vi "32xx_Config_RS232.vi"(4 "Serial_Settings.ctltermination char\n(0xA = '\\n' = LF)":u8=13 format="%x", 6 "Enable Termination\nChar (F)":bool, 7 "Taille buffers E/S":u32=64, 8 "entrée d'erreur":errorcluster caption="entrée d'erreur (pas d'erreur)", 9 "Paramètres série":T1={"Bauds"=9600, "bits"=8, "     Parité :"=enum."None", "bit(s) de stop"=10, "CTRL flux"=0} {"CTRL flux" items=["Aucun(e)"=0, "XON/XOFF"=1, "RTS/CTS"=2, "DTR/DSR"=4]; "bit(s) de stop" items=["1.0"=10, "2.0"=20]; "bits" min=5 max=8 step=1; "Bauds" items=["75"=75, "110"=110, "134"=134, "150"=150, "300"=300, "600"=600, "1200"=1200, "1800"=1800, "2400"=2400, "4800"=4800, "7200"=7200, "9600"=9600, "14400"=14400, "19200"=19200, "28800"=28800, "38400"=38400, "56000"=56000, "57600"=57600, "115200"=115200, "128000"=128000, "230400"=230400]}, 10 "TimeOut (ms)":u32=6500, 11 "Port Entrée":refnum<visa-resource-name>="COM1") -> (0 "sortie d'erreur":errorcluster, 3 "Port Sortie":refnum<visa-resource-name>="COM1")   [LabVIEW 2020]
doc: "Configuration du port COM en RS232 : Baud rate, data bits ; etc.."
panel:
  # "© 2008 2020 elc  ALL RIGHTS RESERVED."
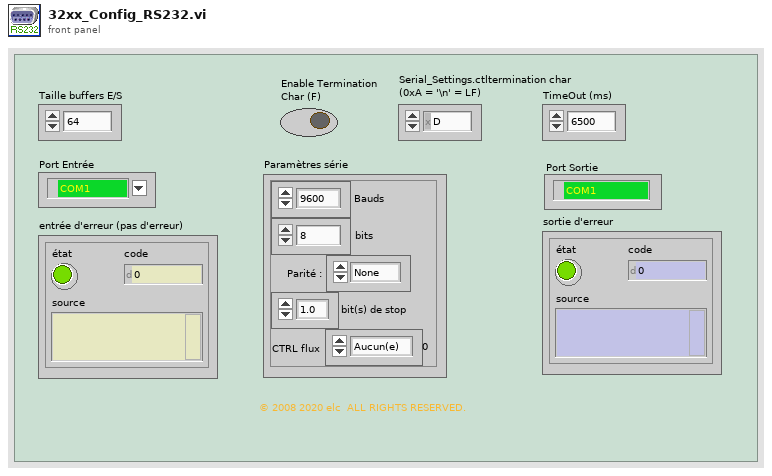
[diagram p1: front panel]
types:
  T1 = cluster{"Bauds":u32, "bits":u16, "     Parité :":enum16{"None", "Odd", "Even", "Mark", "Space"}, "bit(s) de stop":u16, "CTRL flux":u16}
  T2 = typedef "32xx_VISA_Flush_IO_BuffMask_Custom.ctl" = u16
  T3 = typedef "32xx_VISA_Set_IO_Buffer_Mask_Custom.ctl" = u16
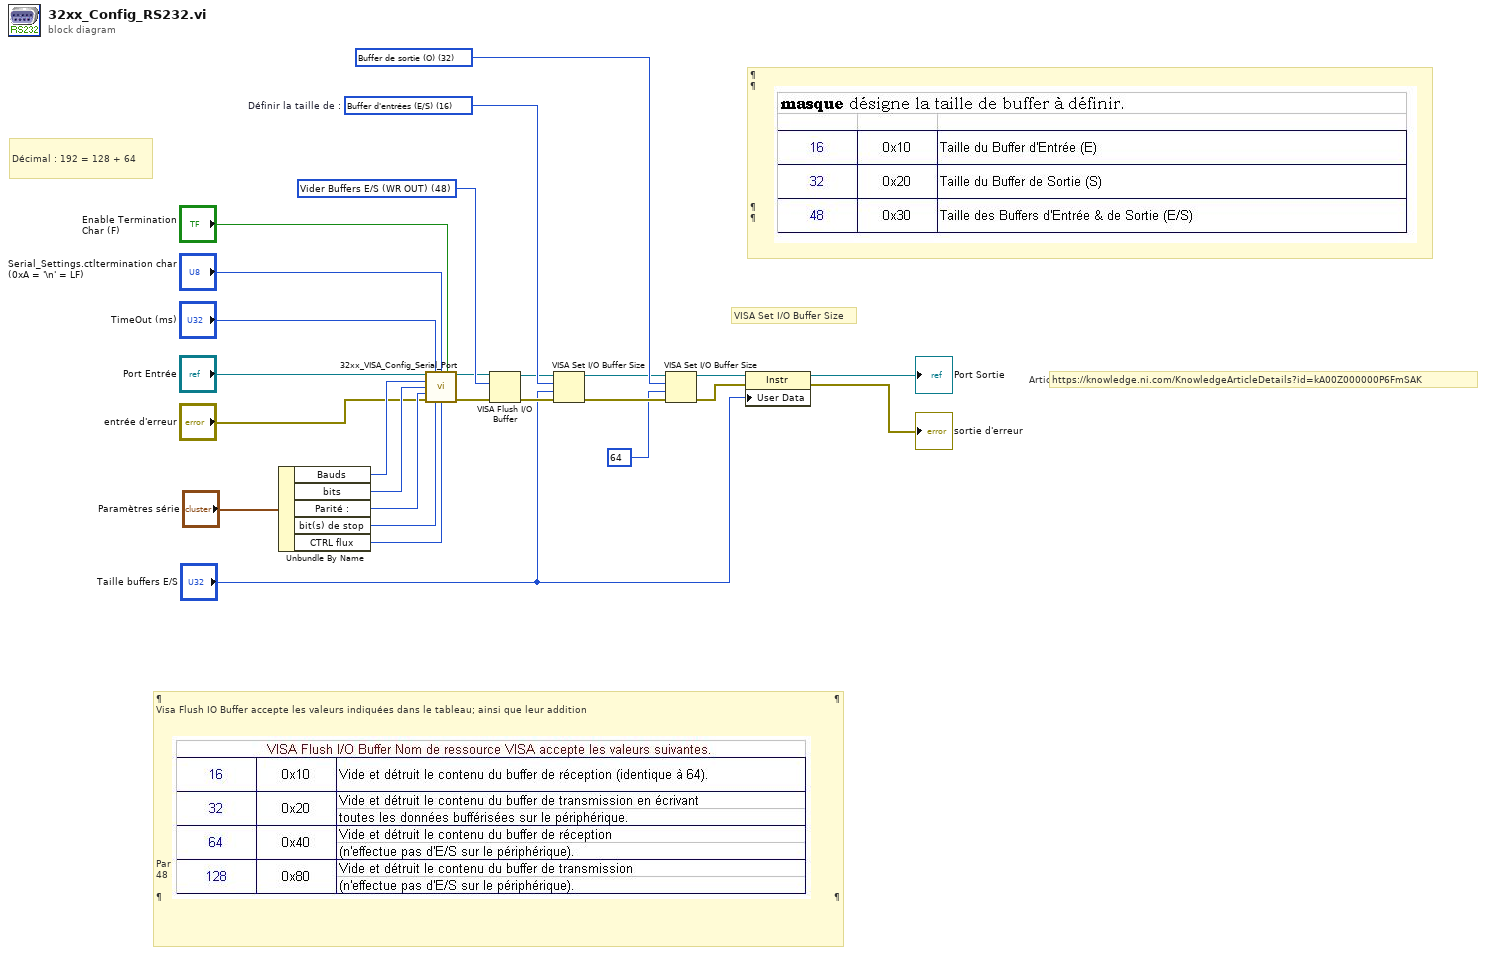
[diagram p0: block diagram]
diagram:
  w19 = T2 48 items=["Vider le buffer d'entrée"=16, "Écrire le buffer de sortie sur le périphérique"=32, "Vider Buffers E/S (WR OUT)"=48, "Vider le buffer d'entrée (Pas d'E/S)"=64, "Vider le buffer de sortie  (sans écrire)"=128, "Vider les buffers E/S  (Pas d'E/S)"=192] ("Mask")
  w22 = T3 32 items=["Buffer d'entrée (I)"=16, "Buffer de sortie (O)"=32, "Buffer d'entrée et de sorties (I/O)"=48] ("Mask")
  w26 = T3 16 items=["Buffer d'entrées (E/S)"=16, "Buffer de sorties (E/S)"=32, "Buffers d'entrées et de sorties (E/S)"=48]  # Définir la taille de :
  # "https://knowledge.ni.com/KnowledgeArticleDetails?id=kA00Z000000P6FmSAK"
  # "Article de labView au sujet  de l'erreur  -1073807298 & du Flush automatique :"
  # "VISA Set I/O Buffer Size"
  # "Décimal : 192 = 128 + 64"
  # "¶                                                                                                                                                                                                                               ¶\n\n\n\n\n\n\n\n\n\n\n¶                                                                                                                                                                                                                               ¶"
  # "¶                                                                                                                                                                                                                                ¶\nVisa Flush IO Buffer accepte les valeurs indiquées dans le tableau; ainsi que leur addition\n\n\n\n\n\n\n\n\n\n\n\n\n\nPar exemple, la valeur 192 (0xC0 = 0x40 + 0x80)  videra les buffers d'entrée & de sortie, sans écrire sur le périphérique.\n48 = 0x30 = 0x10 + 0x20\n\n¶                                                                                                                                                                                                                                ¶"
  n1 = Unbundle By Name("Paramètres série") -> ("Bauds"=w11:u32, "bits"=w10:u16, "Parité :"=w9:enum16{"None", "Odd", "Even", "Mark", "Space"}, "bit(s) de stop"=w4:u16, "CTRL flux"=w3:u16)
  n2 = call "32xx_VISA_Config_Serial_Port.vi"("VISA resource name"="Port Entrée", "timeout (10sec)"="TimeOut (ms)", "termination char\n(0xA = '\\n' = LF)"="Serial_Settings.ctltermination char\n(0xA = '\\n' = LF)", "Enable Termination\nChar (T)"="Enable Termination\nChar (F)", "baud rate (9600)"=w11, "data bits (8)"=w10, "parity (0:none)"=w9, "error in (no error)"="entrée d'erreur", "stop bits (10: 1 bit)"=w4, "flow control (0:none)"=w3) -> ("référence en sortie"=w1:refnum<visa-resource-name>, "error out"=w2:errorcluster)  [unwired: 4 in]
  n3 = VISA Flush I/O Buffer(VISA resource name=w1, mask (16)=w19, error in (no error)=w2) -> (VISA resource name out=w24:refnum<visa-resource-name>, error out=w23:errorcluster)
  n4 = VISA Set I/O Buffer Size(VISA resource name=w24, mask (16)=w26, size (4096)="Taille buffers E/S", error in (no error)=w23) -> (VISA resource name out=w21:refnum<visa-resource-name>, error out=w20:errorcluster)
  n5 = VISA Set I/O Buffer Size(VISA resource name=w21, mask (16)=w22, size (4096)=u32 64 ("taille (4096)"), error in (no error)=w20) -> (VISA resource name out=w17:refnum<visa-resource-name>, error out=w16:errorcluster)
  n6 = property class="Instr"(reference=w17, error in=w16, "User Data"="Taille buffers E/S") -> (reference out=→"Port Sortie":refnum<visa-resource-name>, error out=→"sortie d'erreur":errorcluster)
